vi "kpro.vi"(0 "Output KPRO":path=path "c:/junk.dat", 1 "Initialize":bool, 2 "Finished In":bool, 5 "Absolute Depth In":sgl format="%.2f", 7 "Total Volume in":dbl format="%.2f", 9 "Zeroed Pressure":dbl format="%.2f", 11 "Flow":dbl format="%.2f", 12 "Read String Pot":bool, 13 "Increment":bool, 14 "SS In":i32) -> (4 "Finished Out":bool, 6 "SS Out":i32, 8 "Current Depth Out":sgl format="%.2f", 10 "Total Volume Out":dbl format="%.2f", 15 "Output Array":dbl[][](array[numeric])=[[17182499.0, -1.0, -1.0, 0.07295542423579193, 10.0, 30.0, 1.0, 0.2942041776993234, 33.989999999999995], [17194122.0, -2.0, -2.0, 0.08603630732168976, 10.0, 30.0, 1.0, 0.28579594169762795, 34.989999999999995], [17196835.0, -3.0, -3.0, 0.36859565057132326, 10.0, 30.0, 1.0, 0.27785495971103086, 35.989999999999995], [17198861.0, -4.0, -4.0, 0.493583415597236, 10.0, 30.0, 1.0, 0.27034333603676675, 36.989999999999995], [17203069.0, -5.0, -5.0, 0.23764258555133078, 10.0, 30.0, 1.0, 0.2632271650434325, 37.989999999999995], [17204351.0, -6.0, -6.0, 0.7800312012480499, 10.0, 30.0, 1.0, 0.2564760194921775, 38.989999999999995], [17205734.0, -7.0, -7.0, 0.7230657989877078, 10.0, 30.0, 1.0, 0.25006251562890724, 39.989999999999995], [17206879.0, -8.0, -8.0, 0.8733624454148472, 10.0, 30.0, 1.0, 0.24396194193705784, 40.989999999999995], [17208211.0, -9.0, -9.0, 0.7507507507507507, 10.0, 30.0, 1.0, 0.23815194093831868, 41.989999999999995], [17211804.0, -10.0, -10.0, 0.27831895352073477, 10.0, 30.0, 1.0, 0.23261223540358225, 42.989999999999995], [17214313.0, -11.0, -11.0, 0.3985651654045437, 10.0, 30.0, 1.0, 0.22732439190725168, 43.989999999999995], [17215593.0, -12.0, -12.0, 0.78125, 10.0, 30.0, 1.0, 0.22227161591464772, 44.989999999999995], [17216822.0, -13.0, -13.0, 0.8136696501220504, 10.0, 30.0, 1.0, 0.21743857360295718, 45.989999999999995], [17218103.0, -14.0, -14.0, 0.7806401249024201, 10.0, 30.0, 1.0, 0.2128112364332837, 46.989999999999995], [17219267.0, -15.0, -15.0, 0.859106529209622, 10.0, 30.0, 1.0, 0.20837674515524068, 47.989999999999995], [17220448.0, -16.0, -16.0, 0.8467400508044031, 10.0, 30.0, 1.0, 0.20412329046744235, 48.989999999999995], [17221627.0, -17.0, -17.0, 0.8481764206955046, 10.0, 30.0, 1.0, 0.20004000800160035, 49.989999999999995], [17222775.0, -18.0, -18.0, 0.8710801393728224, 10.0, 30.0, 1.0, 0.19611688566385568, 50.989999999999995], [17223888.0, -19.0, -19.0, 0.8984725965858041, 10.0, 30.0, 1.0, 0.19234468166955185, 51.989999999999995], [17225019.0, -20.0, -20.0, 0.8841732979664014, 10.0, 30.0, 1.0, 0.18871485185884132, 52.989999999999995], [17226151.0, -21.0, -21.0, 0.88339222614841, 10.0, 30.0, 1.0, 0.18521948508983146, 53.989999999999995], [17227282.0, -22.0, -22.0, 0.8841732979664014, 10.0, 30.0, 1.0, 0.18185124568103292, 54.989999999999995]] format="%.5f")   [LabVIEW 2016]
uses:
  Kpro Globals.vi
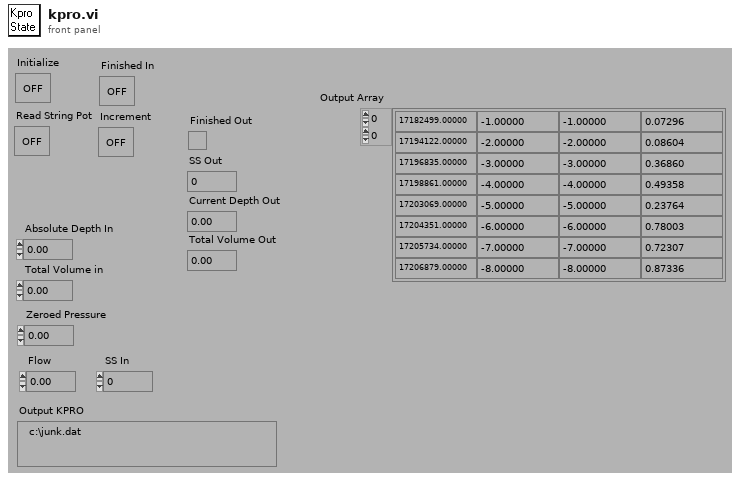
[diagram p1: front panel]
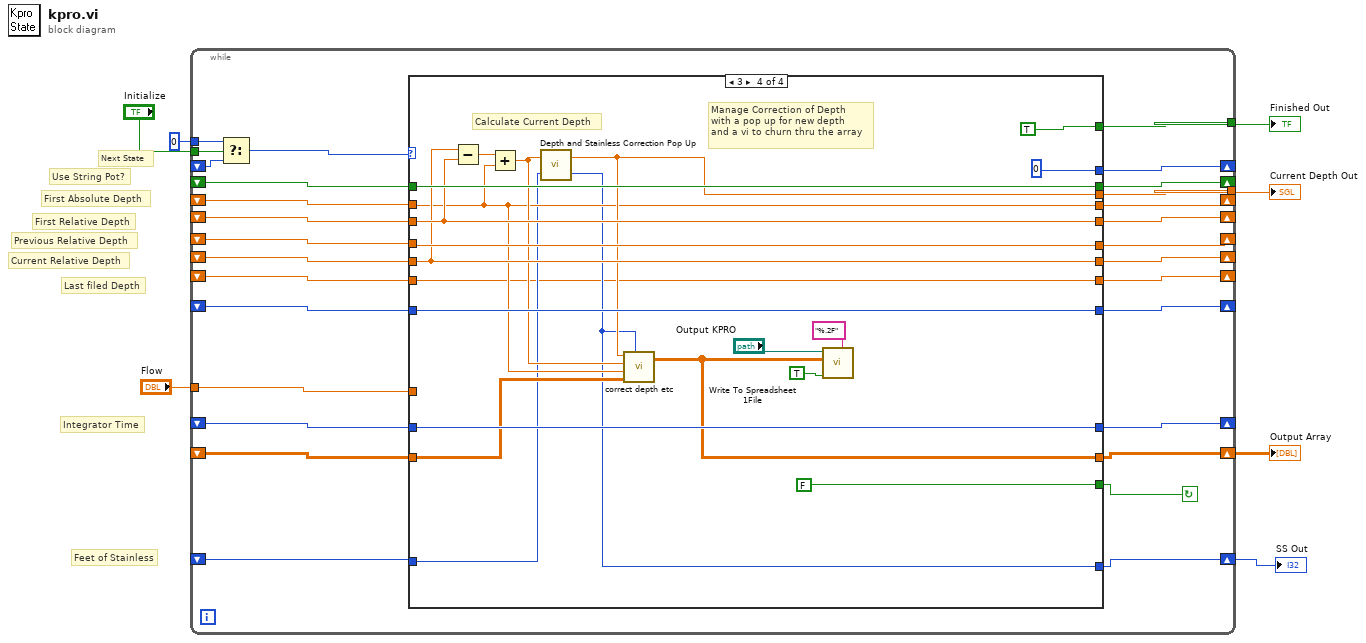
[diagram p0: block diagram]
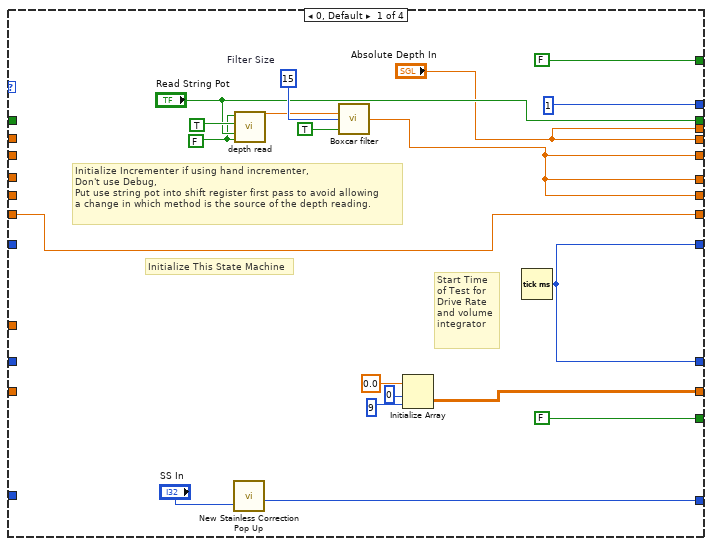
[diagram p2: hidden frame]
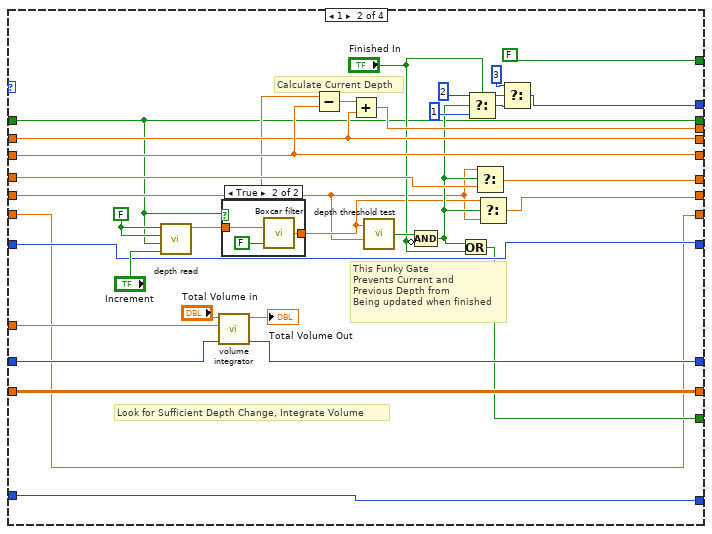
[diagram p3: hidden frame]
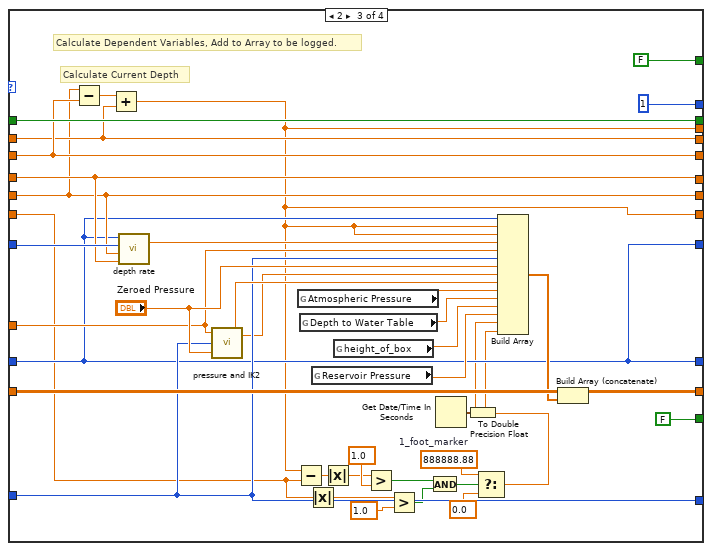
[diagram p5: hidden frame]
diagram:
  # "Last filed Depth"
  # "Feet of Stainless"
  # "Use String Pot?"
  # "Next State"
  # "First Absolute Depth"
  # "Current Relative Depth"
  # "Integrator Time"
  # "Previous Relative Depth"
  # "First Relative Depth"
  n1 = while {
    shift-left: _ -> [w9]
    shift-right: [w10] -> _
    shift-left: _ -> [w12]
    shift-right: [w11] -> w2
    tunnel: [w13] -> w3
    tunnel: [w14] -> w4
    shift-left: _ -> [w15]
    shift-right: [w16] -> _
    shift-left: _ -> [w17]
    shift-right: [w18] -> w1
    shift-left: _ -> [w19]
    shift-right: [w20] -> _
    tunnel: "Flow" -> [w22]
    shift-left: _ -> [w24]
    shift-right: [w25] -> _
    shift-left: _ -> [w23]
    shift-right: [w26] -> _
    shift-left: _ -> [w21]
    shift-right: [w27] -> _
    shift-left: _ -> [w28]
    shift-right: [w29] -> _
    shift-left: _ -> [w30]
    shift-right: [w31] -> _
    tunnel: "Initialize" -> [w33]
    tunnel: 0 -> [w34]
    shift-left: _ -> [w36]
    shift-right: [w32] -> _
    stop <- w8 continue-if-true
    n2 = Select(t=w34, s=w33, f=w36) -> (s? t:f=w35:i32)
    n3 = case shown="3" w35 {
      tunnel: [1 w79 1 0] -> w32
      tunnel: [w47 w71 w120 w144] -> w31
      tunnel: w30 -> [_ w71 w120 w144]
      tunnel: ["Read String Pot" w57 w129 w148] -> w29
      tunnel: w28 -> [_ w57 w129 w148]
      tunnel: [w48 w80 w107 w149] -> w27
      tunnel: [w48 w73 w107 w150] -> w26
      tunnel: [w47 w84 w123 w146] -> w25
      tunnel: w24 -> [_ w67 w123 w146]
      tunnel: w23 -> [_ w74 w107 w150]
      tunnel: w22 -> [_ w72 w113 _]
      tunnel: w21 -> [_ w80 w124 w149]
      tunnel: [w47 w66 w116 w143] -> w20
      tunnel: w19 -> [_ w58 w116 w143]
      tunnel: [w46 w81 w126 w137] -> w18
      tunnel: w17 -> [_ w81 w127 w142]
      tunnel: ["Absolute Depth In" w69 w119 w139] -> w16
      tunnel: w15 -> [_ w69 w119 w139]
      tunnel: ["Absolute Depth In" w68 w105 w140] -> w14
      tunnel: [FALSE w64 FALSE FALSE] -> w8
      tunnel: [FALSE FALSE FALSE TRUE] -> w13
      tunnel: w12 -> [_ w60 w114 w133]
      tunnel: [w38 w60 w114 w132] -> w11
      tunnel: [w37 w56 w105 w131] -> w10
      tunnel: w9 -> [w37 w56 w95 w131]
      frame 0, Default {
        w49 = FALSE
        w53 = 15  # Filter Size
        # "Initialize This State Machine"
        # "Start Time\nof Test for\nDrive Rate\nand volume\nintegrator"
        # "Initialize Incrementer if using hand incrementer,\nDon't use Debug,\nPut use string pot into shift register first pass to avoid allowing\na change in which method is the source of the depth reading."
        n4 = call "New Stainless Correction Pop Up.vi"("New Feet\n of Stainless\n(Count)"="SS In") -> ("Feet of\nStainless to be\nUsed (Count)"=w38:i32)  [unwired: 2 in]
        n5 = call "depth read.vi"("Increment Button"=w49, "Read String Pot"="Read String Pot", "Initialize Debug"=TRUE, "Debug"=w49) -> ("Distance"=w52:dbl)
        n6 = call "Boxcar filter.vi"("Initialize"=TRUE, "Filter Size"=w53, "Filter Input"=w52) -> ("Filter Output"=w47:dbl)
        n7 = Initialize Array(0.0, 0, 9) -> (w46:dbl[][])
        n8 = Tick Count (ms)() -> (millisecond timer value=w48:u32)
      }
      frame 1 {
        w86 = FALSE
        # "This Funky Gate\nPrevents Current and \nPrevious Depth from \nBeing updated when finished"
        # "Look for Sufficient Depth Change, Integrate Volume"
        # "Calculate Current Depth"
        n9 = call "depth read.vi"("Increment Button"="Increment", "Read String Pot"=w57, "Initialize Debug"=w86, "Debug"=w86) -> ("Distance"=w87:dbl)
        n10 = call "volume integrator.vi"("Previous Time (msec)"=w74, "Flow"=w72, "Total Volume in"="Total Volume in") -> ("Current Time (msec)"=w73:u32, "Total Volume Out"=→"Total Volume Out":dbl)  [unwired: 3 in]
        n11 = case shown="True" w57 {
          tunnel: w87 -> [w88 w90]
          tunnel: [w88 w89] -> w59
          frame False {
          }
          frame True {
            n12 = call "Boxcar filter.vi"("Initialize"=FALSE, "Filter Input"=w90) -> ("Filter Output"=w89:dbl)  [unwired: 1 in]
          }
        }
        n13 = Subtract(x=w58, y=w71) -> (x-y=w70:dbl)
        n14 = Add(x=w70, y=w69) -> (x+y=w68:dbl)
        n15 = call "depth threshold test.vi"("Depth\nPrevious"=w58, "Depth \nCurrent"=w59) -> ("Threshold\nExceeded"=w65:bool)
        n16 = Compound Arithmetic op=AND(w65, invert "Finished In") -> (w63:bool)
        n17 = Or(x=w63, y="Finished In") -> (x .or. y?=w64:bool)
        n18 = Select(t=2, s=w63, f=1) -> (s? t:f=w78:i32)
        n19 = Select(t=w58, s=w63, f=w67) -> (s? t:f=w84:dbl)
        n20 = Select(t=w59, s=w63, f=w58) -> (s? t:f=w66:dbl)
        n21 = Select(t=3, s="Finished In", f=w78) -> (s? t:f=w79:i32)
      }
      frame 2 {
        w101 = 888888.88  # 1_foot_marker
        # "Calculate Dependent Variables, Add to Array to be logged."
        # "Calculate Current Depth"
        n22 = Subtract(x=w116, y=w120) -> (x-y=w121:dbl)
        n23 = Add(x=w121, y=w119) -> (x+y=w105:dbl)
        n24 = call "depth rate.vi"("Depth Last"=w123, "Depth Current"=w116, "Time Last"=w124, "Time Current"=w107) -> ("Depth Rate"=w122:dbl)
        n25 = call "pressure and IK2.vi"("Pressure"="Zeroed Pressure", "Ft. of SS"=w114, "flow"=w113) -> ("Corrected Headloss"=w128:dbl, "IK"=w112:dbl)
        n26 = Subtract(x=w105, y=w95) -> (x-y=w104:dbl)
        n27 = global read "Kpro Globals.vi" "Atmospheric Pressure"() -> (w111:dbl)
        n28 = global read "Kpro Globals.vi" "Depth to Water Table"() -> (w109:dbl)
        n29 = Absolute Value(x=w95) -> (abs(x)=w93:dbl)
        n30 = global read "Kpro Globals.vi" "Reservoir Pressure"() -> (w110:dbl)
        n31 = Absolute Value(x=w104) -> (abs(x)=w102:dbl)
        n32 = global read "Kpro Globals.vi" "height_of_box"() -> (w108:dbl)
        n33 = Greater?(x=w102, y=1.0) -> (0:w97:bool)
        n34 = Greater?(x=w93, y=1.0) -> (0:w96:bool)
        n35 = And(x=w97, y=w96) -> (x .and. y?=w98:bool)
        n36 = Get Date/Time In Seconds() -> (seconds since 1Jan1904=w92:timestamp)
        n37 = To Double Precision Float(number=w92) -> (double precision float=w106:dbl)
        n38 = Select(t=w101, s=w98, f=0.0) -> (s? t:f=w99:dbl)
        n39 = Build Array(w107, w105, w105, w122, w113, w114, "Zeroed Pressure", w112, w128, w111, w109, w108, w110, w106, w99) -> (w125:dbl[])
        n40 = Build Array (concatenate)(w127, w125) -> (w126:dbl[][])
      }
      frame 3 {
        # "Manage Correction of Depth\nwith a pop up for new depth\nand a vi to churn thru the array"
        # "Calculate Current Depth"
        n41 = Subtract(x=w143, y=w144) -> (x-y=w145:dbl)
        n42 = Add(x=w145, y=w139) -> (x+y=w141:dbl)
        n43 = call "Depth and Stainless Correction Pop Up.vi"("New Number\n of Stainless\n(Count)"=w133, "Input \nCorrected \nDepth (Feet)"=w141) -> ("Feet of\nStainless to be\nUsed (Count)"=w132:i32, "Depth to \nbe Used \n(Feet)"=w140:sgl)
        n44 = call "correct depth etc.vi"("Correct Depth"=w140, "Incorrect Depth"=w141, "First Absolute Depth"=w139, "Uncorrected Array"=w142, "New Stainless Feet"=w132) -> ("Corrected Array"=w137:dbl[][])  [unwired: 1 in]
        n45 = call "Write To Spreadsheet 1File.vi"("format (%.3f)"="%.2F", "append to file? (new file:F)"=TRUE, "2D data"=w137, "file path (dialog if empty)"="Output KPRO") -> ()  [unwired: 4 in, 1 out]
      }
    }
  }
  "Current Depth Out" <- w4
  "Finished Out" <- w3
  "SS Out" <- w2
  "Output Array" <- w1
